vi "_TestExec.TEST Health Indicator State Controller.vi"() -> ()   [LabVIEW 2018]
panel:
  in  "Warnings In":i32 caption="Counts"
  in  "Errors In":i32 caption="Errors"
  out "Health OK":bool
  out "Errors":i32
  out "Warnings":i32 caption="Counts"
  in  "Go to Health Details":bool
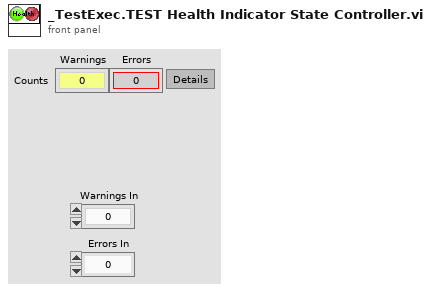
[diagram p1: front panel]
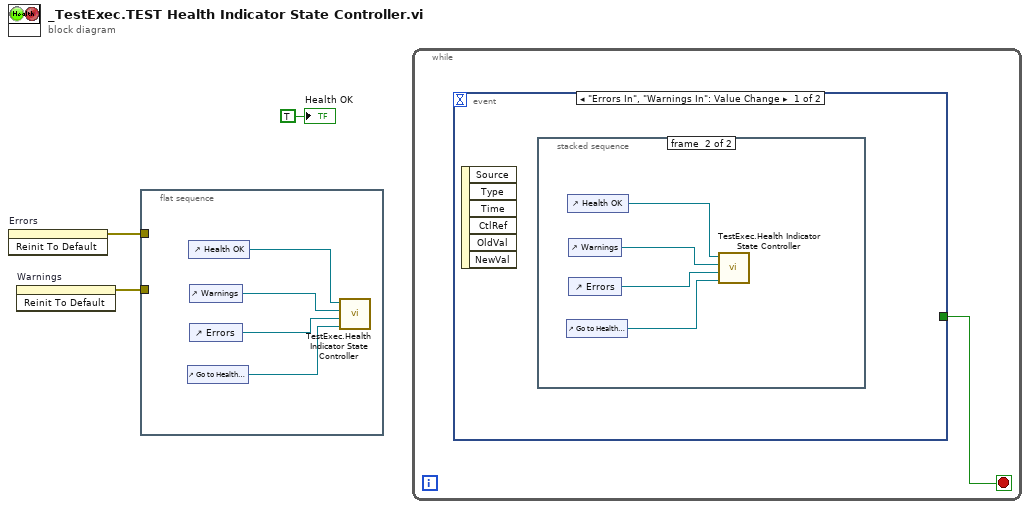
[diagram p0: block diagram]
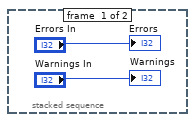
[diagram p2: hidden frame]
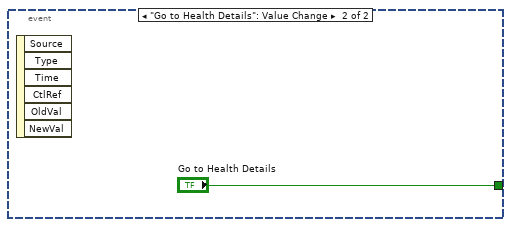
[diagram p3: hidden frame]
diagram:
  n1 = invoke on="Errors" class="DigNum (strict)" method="Reinit To Default"() -> (error out=w2:errorcluster)  [unwired: 3 in, 2 out]
  n2 = invoke on="Warnings" class="DigNum (strict)" method="Reinit To Default"() -> (error out=w1:errorcluster)  [unwired: 3 in, 2 out]
  n3 = flat-sequence {
    tunnel: w2 -> [_]
    tunnel: w1 -> [_]
    frame #0 {
      n4 = control-ref of="Go to Health Details"() -> (w7:refnum<vi>)
      n5 = control-ref of="Health OK"() -> (w4:refnum<vi>)
      n6 = control-ref of="Warnings"() -> (w5:refnum<vi>)
      n7 = control-ref of="Errors"() -> (w6:refnum<vi>)
      n8 = call "TestExec.Health Indicator State Controller.vi"("Go to Details"=w7, "Errors Cntr"=w6, "Warnings Cntr"=w5, "Health Bool"=w4) -> ()  [unwired: 8 in]
    }
  }
  n9 = while {
    stop <- w8 stop-if-true
    n10 = event shown="[0] \"Errors In\", \"Warnings In\": Value Change" {
      selector: _ -> [_ _]
      dyn-events: _ -> [_ _]
      timeout: _ -> [_ _]
      tunnel: [_ "Go to Health Details"] -> w8
      event "Errors In", "Warnings In": Value Change {
        n11 = event-data() -> ()  [unwired: 1 in, 6 out]
        n12 = stacked-sequence {
          frame #0 {
            "Warnings" <- "Warnings In"
            "Errors" <- "Errors In"
          }
          frame #1 {
            n13 = control-ref of="Go to Health Details"() -> (w11:refnum<vi>)
            n14 = control-ref of="Health OK"() -> (w14:refnum<vi>)
            n15 = control-ref of="Warnings"() -> (w13:refnum<vi>)
            n16 = control-ref of="Errors"() -> (w12:refnum<vi>)
            n17 = call "TestExec.Health Indicator State Controller.vi"("Go to Details"=w11, "Errors Cntr"=w12, "Warnings Cntr"=w13, "Health Bool"=w14) -> ()  [unwired: 8 in]
          }
        }
      }
      event "Go to Health Details": Value Change {
        n18 = event-data() -> ()  [unwired: 1 in, 6 out]
      }
    }
  }
  "Health OK" <- TRUE ("Health OK")
